vi "goToHome.vi"(0 "SingleAxisController in":refnum<class "_SingleAxisController.lvclass">, 1 "axis (nc - for multi-axis applications only)":T2, 2 "dir":T1, 3 "mode (nc - for multi-axis applications only)":T3, 5 "error in (no error)":errorcluster) -> (14 "SingleAxisController out":refnum<class "_SingleAxisController.lvclass">, 17 "success?":bool, 18 "response":string, 19 "error out":errorcluster)   [LabVIEW 2013, in "classes.lvlib" / "_SingleAxisController.lvclass"]
doc: "Produced By:\n\n<B>Kod Integrations, LLC</B>\n4835 Marianne Drive\nMount Airy, MD 21771\nhttp://www.kodintegrations.com\nemail: info@kodintegrations.com\nphone: (240) 687-1288"
uses:
  _SingleAxisController.lvclass
  common/controls/homing_mode.ctl
  common/controls/axis.ctl
  common/controls/linear_direction.ctl
  Controller/_Controller.lvclass
  libraries/common.lvlib
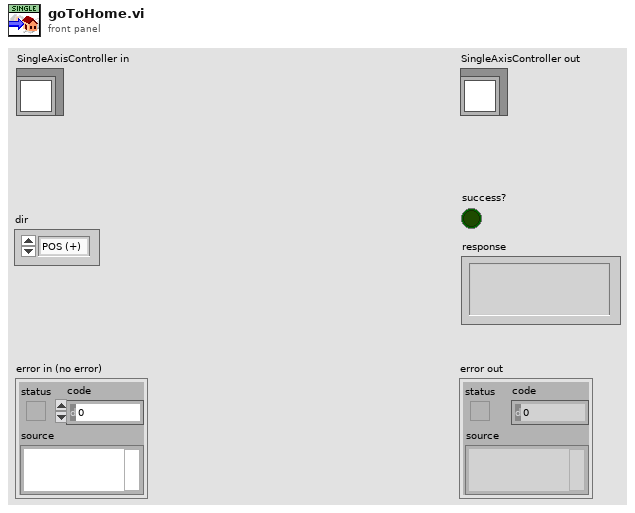
[diagram p1: front panel]
types:
  T1 = typedef "common.lvlib/linear_direction.ctl" = enum16{"POS (+)", "NEG (-)"}
  T2 = typedef "common.lvlib/axis.ctl" = enum16{"X", "Y", "Z", "U"}
  T3 = typedef "common.lvlib/homing_mode.ctl" = enum16{"HOME_INPUT (HIGH SPEED)", "LIMIT_INPUT", "HOME_INPUT_&_Z-INDEX", "Z-INDEX", "HOME_INPUT (HIGH_&_LOW_SPEED)"}
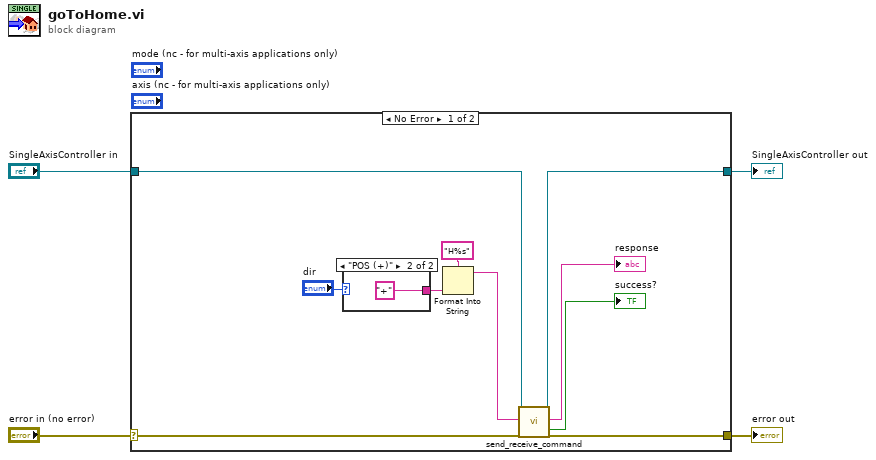
[diagram p0: block diagram]
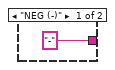
[diagram p2: hidden frame]
diagram:
  n1 = case shown="No Error" "error in (no error)" {
    selector: "error in (no error)" -> [w11 w18]
    tunnel: [w10 w18] -> w3
    tunnel: [w6 w17] -> w1
    tunnel: "SingleAxisController in" -> [w7 w17]
    frame No Error {
      n2 = case shown="\"POS (+)\"" "dir" {
        tunnel: ["-" "+"] -> w13
        frame "NEG (-)" {
        }
        frame "POS (+)" {
        }
      }
      n3 = Format Into String(format string="H%s", w13) -> (resulting string=w12:string)  [unwired: 2 in, 1 out]
      n4 = call "send_receive_command.vi"("reference (in)"=w7, "ASCII Command (in)"=w12, "error in (no error)"=w11) -> ("reference (out)"=w6:refnum<class "_SingleAxisController.lvclass">, "response (out)"=→"response":string, "success?"=→"success?":bool, "error out"=w10:errorcluster)  [unwired: 12 in, 1 out]
    }
    frame Error {
    }
  }
  "error out" <- w3
  "SingleAxisController out" <- w1
